vi "algo.test.add.two.buys.prepend.vi"() -> ()   [LabVIEW 2020]
uses:
  types/val.algo.pretty.watchlist.ctl
  common/types/val.pretty.orderbook.ctl
panel:
  in  "Value":u64=165 format="%.0x"
  in  "exp.OrderBooks.out":T1[](array[typedef])=[{"metadata"={"Symbol"="AAPL", "# of Buys"=2, "# of Sells"=0}, "Bid (Buy)"=[{"OrderId"=50, "Price"=100.35}, {"OrderId"=49, "Price"=100.2}], "Ask (Sell)"=[]}] {"Ask (Sell)"."OrderId" format="%.0x"; "Bid (Buy)"."OrderId" format="%.0x"}
  out "Debug.out":T2(array[cluster]) {"Numeric" format="%.0x"; "Numeric" format="%.0x"}
  out "OrderBooks.out":T1[](array[typedef]) {"Ask (Sell)"."OrderId" format="%.0x"; "Bid (Buy)"."OrderId" format="%.0x"}
  in  "Watchlist":T3[](array[typedef])=[{"symbol"="AAPL", "buy.start.addr"=0, "buy.size"=0, "buy.slots"=100, "sell.start.addr"=100, "sell.size"=0, "sell.slots"=100, "min.ask"=100.25, "max.bid"=1000.5}] {"max.bid" format="%.2f"; "min.ask" format="%.2f"}
  in  "Type, Side, OrderId, Quantity, Symbol, Price, ExeQty, CancelQty, RemQty, Seconds, Nanoseconds, Add, Edit, Remove":string="AddOrder, Buy, 0x31, 100, AAPL, 100.20, 0, 0, 0, 0, 0, True, False, False\nAddOrder, Buy, 0x32, 100, AAPL, 100.35, 0, 0, 0, 0, 0, True, False, False"
  out "Passed":bool
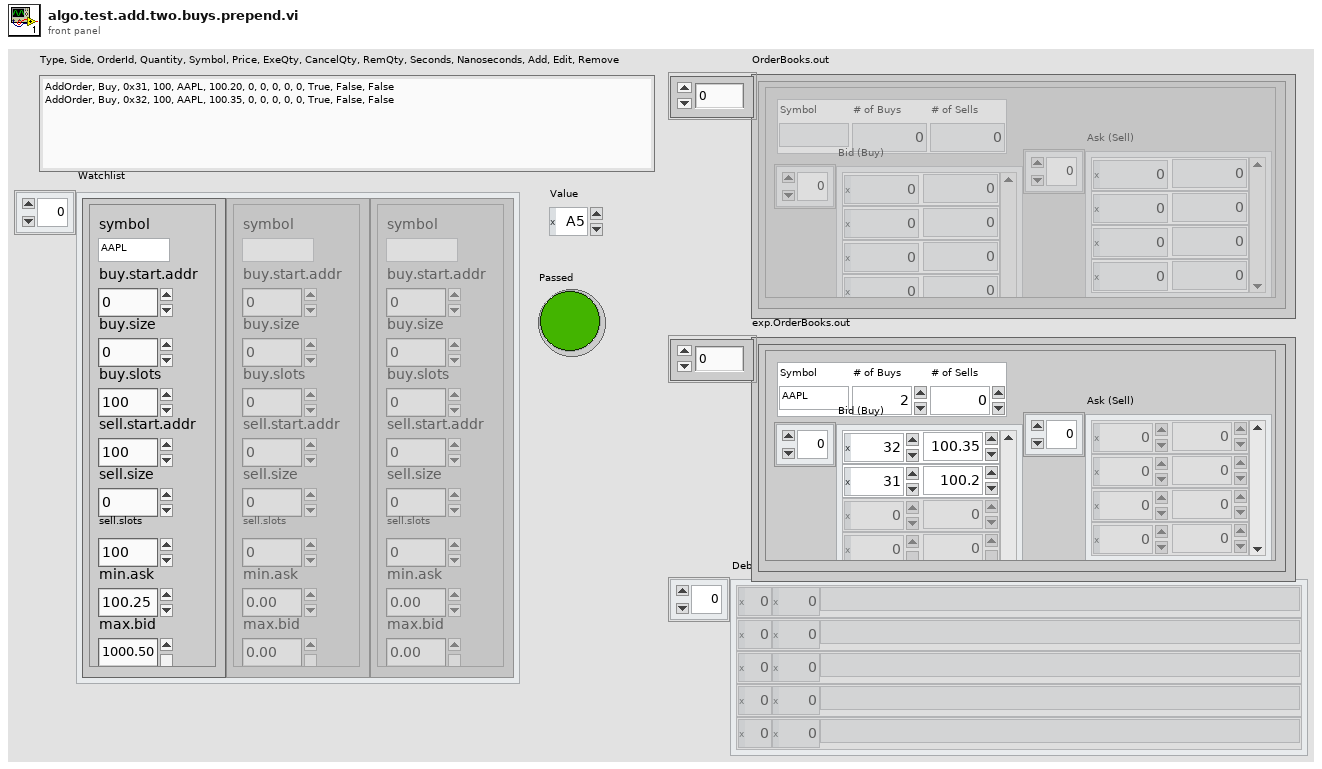
[diagram p1: front panel]
types:
  T1 = typedef "val.pretty.orderbook.ctl" = cluster{"metadata":cluster{"Symbol":string, "# of Buys":u64, "# of Sells":u64}, "Bid (Buy)":cluster{"OrderId":u64, "Price":dbl}[], "Ask (Sell)":cluster{"OrderId":u64, "Price":dbl}[]}
  T2 = cluster{"Numeric":u64, "Numeric":u64, "String":string}[]
  T3 = typedef "val.algo.pretty.watchlist.ctl" = cluster{"symbol":string, "buy.start.addr":u16, "buy.size":u16, "buy.slots":u16, "sell.start.addr":u16, "sell.size":u16, "sell.slots":u16, "min.ask":dbl, "max.bid":dbl}
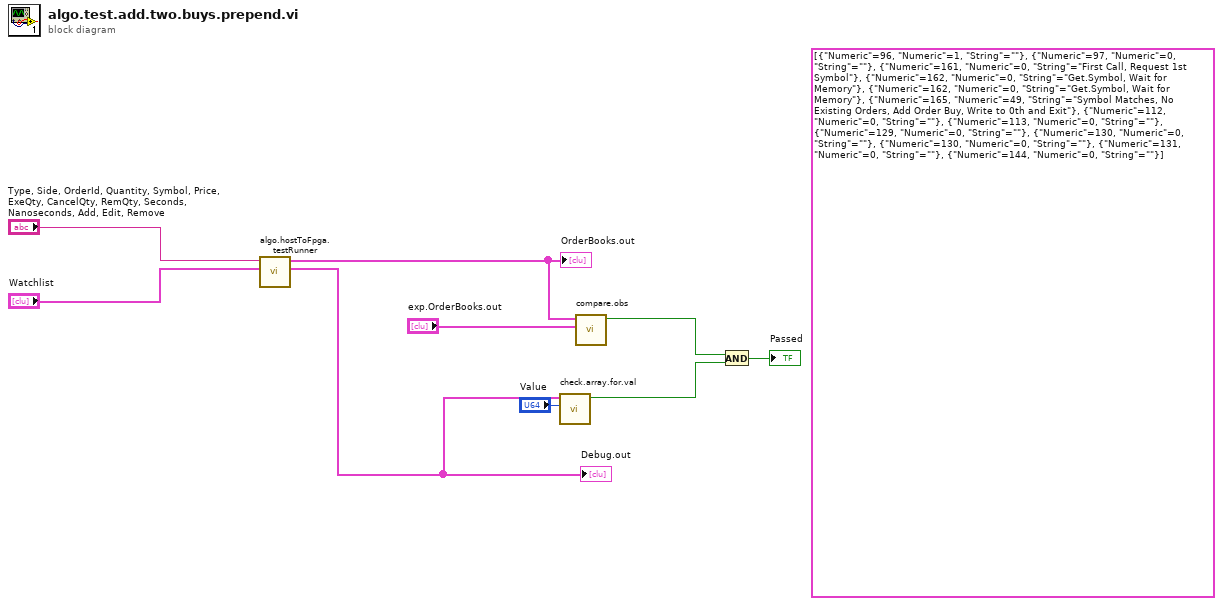
[diagram p0: block diagram]
diagram:
  (unwired) T2 [{"Numeric"=96, "Numeric"=1, "String"=""}, {"Numeric"=97, "Numeric"=0, "String"=""}, {"Numeric"=161, "Numeric"=0, "String"="First Call, Request 1st Symbol"}, {"Numeric"=162, "Numeric"=0, "String"="Get.Symbol, Wait for Memory"}, {"Numeric"=162, "Numeric"=0, "String"="Get.Symbol, Wait for Memory"}, {"Numeric"=165, "Numeric"=49, "String"="Symbol Matches, No Existing Orders, Add Order Buy, Write to 0th and Exit"}, {"Numeric"=112, "Numeric"=0, "String"=""}, {"Numeric"=113, "Numeric"=0, "String"=""}, {"Numeric"=129, "Numeric"=0, "String"=""}, {"Numeric"=130, "Numeric"=0, "String"=""}, {"Numeric"=130, "Numeric"=0, "String"=""}, {"Numeric"=131, "Numeric"=0, "String"=""}, {"Numeric"=144, "Numeric"=0, "String"=""}] ("Debug.out")
  n1 = call "algo.hostToFpga.testRunner.vi"("Watchlist"="Watchlist", "Commands.In (Json)"="Type, Side, OrderId, Quantity, Symbol, Price, ExeQty, CancelQty, RemQty, Seconds, Nanoseconds, Add, Edit, Remove") -> ("Debug.out"=w5:T2, "OrderBooks.out"=w7:T1[])  [unwired: 7 in, 1 out]
  "OrderBooks.out" <- w7
  "Debug.out" <- w5
  n2 = call "check.array.for.val.vi"("Value"="Value", "Debug.in"=w5) -> ("Passed"=w2:bool)  [unwired: 9 in]
  n3 = call "compare.obs.vi"("expected.OrderBooks.out"="exp.OrderBooks.out", "actual.OrderBooks.out"=w7) -> ("Passed"=w3:bool)  [unwired: 8 in, 1 out]
  n4 = And(x=w3, y=w2) -> (x .and. y?=→"Passed":bool)
